vi "Get Signal Units All.vi"(8 "error in":errorcluster) -> (0 "error out":errorcluster, 3 "Signal Units":string[](array[string]))   [LabVIEW 2021, in "XNET-CAN-Signal-Logger.lvlib"]
uses:
  XNET-CAN-Signal-Logger.lvlib
  Global Variables.vi
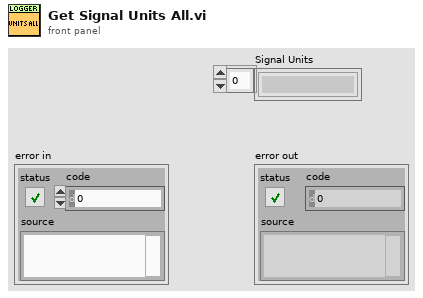
[diagram p1: front panel]
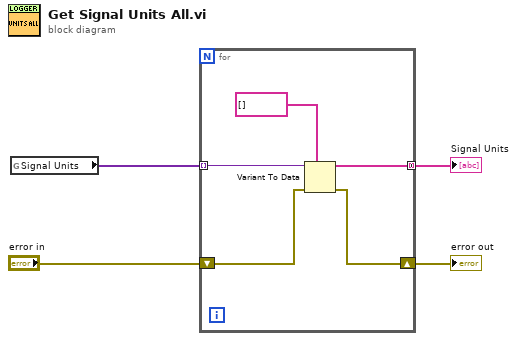
[diagram p0: block diagram]
diagram:
  n1 = global read "Global Variables.vi" "Signal Units"() -> (w4:variant[])
  n2 = for {
    tunnel: w4 -> [w9] mode=indexing
    tunnel: [w7] -> w3 mode=concatenating
    shift-right: [w5] -> w1
    shift-left: "error in" -> [w6]
    n3 = Variant To Data(error in=w6, type=string[] [], Variant=w9) -> (data=w7:string[], error out=w5:errorcluster)
  }
  "Signal Units" <- w3
  "error out" <- w1
